vi "Init Tree.vi"(10 "Settings In":T4={"Step Values"=[], "Only Execute When Test Running"=TRUE, "Reset Sequence When Test Starts"=TRUE, "Current Sequence ID"=0, "Total Iterations"=0, "Current Step Start Timestamp"=0.0, "Number of Sequence Steps"=0, "Num of Analog Channels"=0, "Num of Digital Channels"=0, "Delay Before Starting Sequence"=0.0, "Show UI"=FALSE, "Time Remaining"=0.0, "Test Running"=FALSE, "Pause Timestamp"=0.0}, 11 "Init Refs":T3) -> (2 "Tree Data":cluster{string[], T1[]} {"?"."Data Type" items=["Tree Parent"=-1, "Numeric"=0, "String"=1, "Boolean"=2, "Enum"=3]}, 3 "Selected Tag":string)   [LabVIEW 2020, in "Sequencer with Output Values.lvlib" / "Sequencer with Output Values.lvclass"]
uses:
  Sequencer with Output Values.lvclass
  Params.ctl
  Step Settings.ctl
  Control Refs.ctl
  Tree Item Settings.ctl
  Data Type.ctl
  Global Tree Data.vi
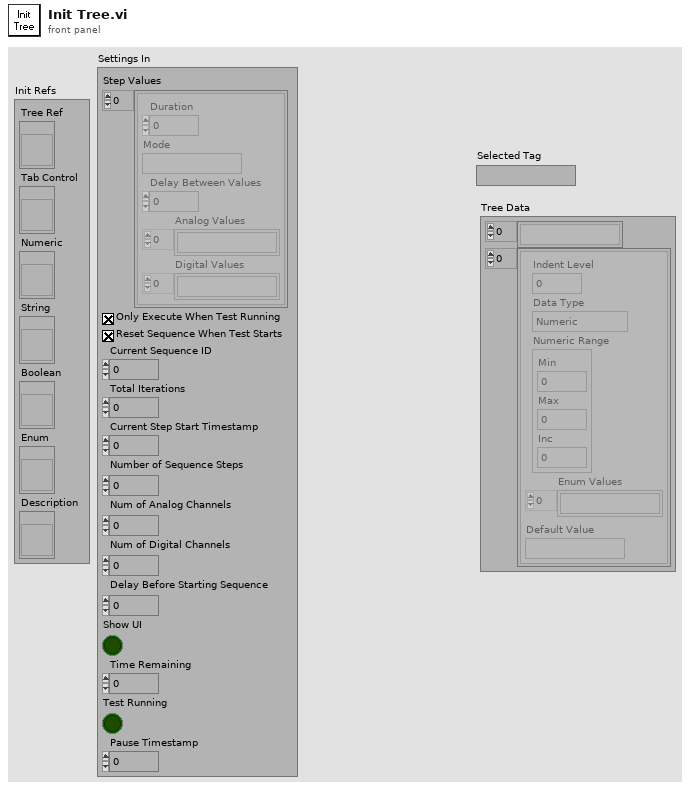
[diagram p1: front panel]
types:
  T1 = typedef "Sequencer with Output Values.lvlib/Sequencer with Output Values.lvclass/Tree Item Settings.ctl" = cluster{"Indent Level":i32, "Data Type":T2, "Numeric Range":cluster{"Min":dbl, "Max":dbl, "Inc":dbl}, "Enum Values":string[], "Default Value":string}
  T2 = typedef "Sequencer with Output Values.lvlib/Sequencer with Output Values.lvclass/Data Type.ctl" = i16
  T3 = typedef "Sequencer with Output Values.lvlib/Sequencer with Output Values.lvclass/Control Refs.ctl" = cluster{"Tree Ref":refnum<vi>, "Tab Control":refnum<vi>, "Numeric":refnum<vi>, "String":refnum<vi>, "Boolean":refnum<vi>, "Enum":refnum<vi>, "Description":refnum<vi>}
  T4 = typedef "Sequencer with Output Values.lvlib/Sequencer with Output Values.lvclass/Params.ctl" = cluster{"Step Values":T5[], "Only Execute When Test Running":bool, "Reset Sequence When Test Starts":bool, "Current Sequence ID":u32, "Total Iterations":u32, "Current Step Start Timestamp":dbl, "Number of Sequence Steps":i32, "Num of Analog Channels":i32, "Num of Digital Channels":i32, "Delay Before Starting Sequence":dbl, "Show UI":bool, "Time Remaining":dbl, "Test Running":bool, "Pause Timestamp":dbl}
  T5 = typedef "Sequencer with Output Values.lvlib/Sequencer with Output Values.lvclass/Step Settings.ctl" = cluster{"Duration":dbl, "Mode":string, "Delay Between Values":dbl, "Analog Values":string[], "Digital Values":string[]}
  T6 = cluster{"Left Cell String":string, "Child Text":string[], "Child Tag":string, "Item Indent":i32, "Child Only?":bool, "Glyph Index":i32}
  T7 = cluster{"Left Cell String":string, "Child Text":string[], "Child Tag":string, "Item Indent":i32, "Child Only?":bool, "Glyph Index":i32}[]
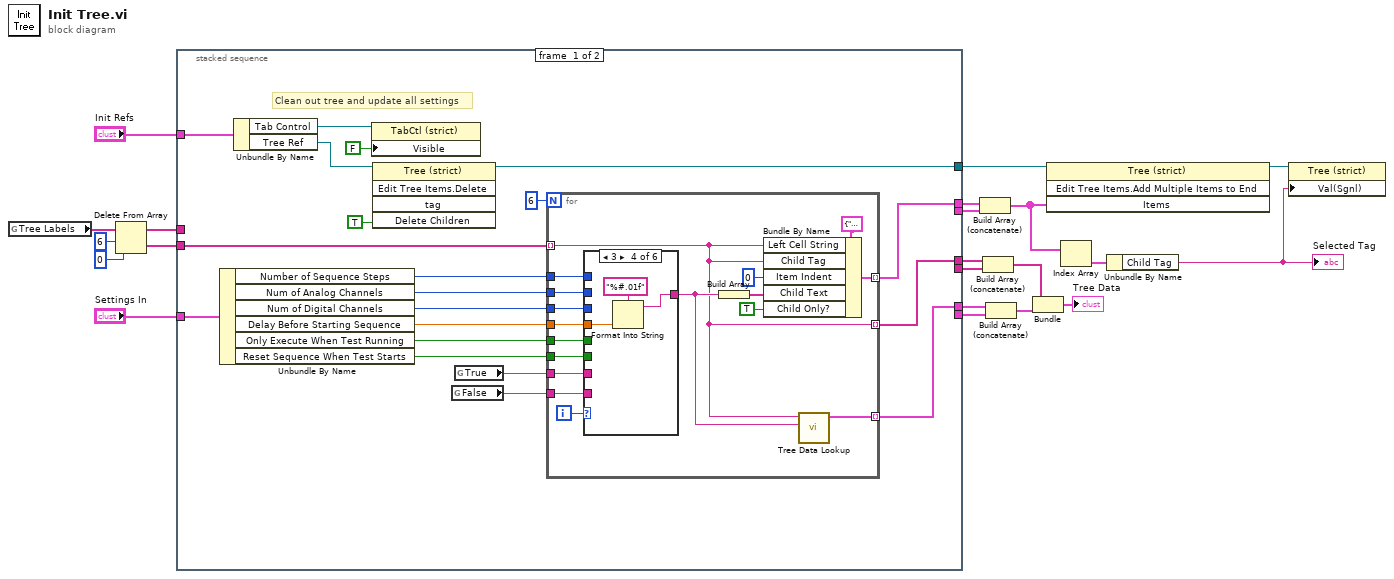
[diagram p0: block diagram]
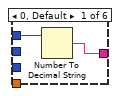
[diagram p2: hidden frame]
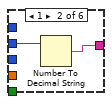
[diagram p3: hidden frame]
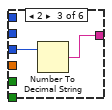
[diagram p4: hidden frame]
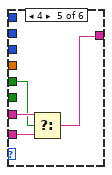
[diagram p5: hidden frame]
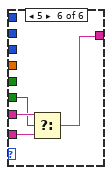
[diagram p6: hidden frame]
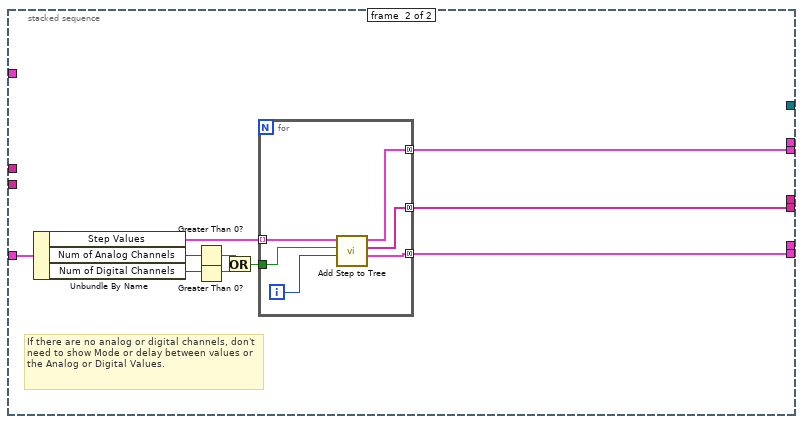
[diagram p7: hidden frame]
diagram:
  n1 = global read "Global Tree Data.vi" "Tree Labels"() -> (w16:string[])
  n2 = Delete From Array(array=w16, length=6, index=0) -> (deleted portion=w13:string[], array with subset deleted=w12:string[])
  n3 = stacked-sequence {
    tunnel: "Init Refs" -> [w39 _]
    tunnel: "Settings In" -> [w36 w85]
    tunnel: [_ w81] -> w18
    tunnel: [w26 _] -> w19
    tunnel: [w25 _] -> w17
    tunnel: w13 -> [w24 _]
    tunnel: w12 -> [_ _]
    tunnel: [w23 _] -> w7
    tunnel: [w22 _] -> w5
    tunnel: [_ w80] -> w2
    tunnel: [_ w79] -> w1
    frame #0 {
      # "Clean out tree and update all settings"
      n4 = Unbundle By Name(w36) -> ("Number of Sequence Steps"=w34:i32, "Num of Analog Channels"=w33:i32, "Num of Digital Channels"=w32:i32, "Delay Before Starting Sequence"=w31:dbl, "Only Execute When Test Running"=w30:bool, "Reset Sequence When Test Starts"=w29:bool)
      n5 = Unbundle By Name(w39) -> ("Tab Control"=w38:refnum<vi>, "Tree Ref"=w41:refnum<vi>)
      n6 = property class="TabCtl (strict)"(reference=w38, "Visible"=FALSE) -> ()  [unwired: 1 in, 2 out]
      n7 = invoke class="Tree (strict)" method="Edit Tree Items.Delete"(reference=w41, "Delete Children"=TRUE ("Delete Children?")) -> (reference out=w25:refnum<vi>)  [unwired: 3 in, 4 out]
      n8 = global read "Global Tree Data.vi" "False"() -> (w27:string)
      n9 = global read "Global Tree Data.vi" "True"() -> (w28:string)
      n10 = for {
        N: 6 -> [_]
        tunnel: w24 -> [w42] mode=indexing
        tunnel: w34 -> [w56]
        tunnel: w33 -> [w55]
        tunnel: w32 -> [w54]
        tunnel: w31 -> [w53]
        tunnel: w30 -> [w52]
        tunnel: w29 -> [w51]
        tunnel: w28 -> [w48]
        tunnel: w27 -> [w47]
        tunnel: [w46] -> w26 mode=indexing
        tunnel: [w43] -> w23 mode=indexing
        tunnel: [w42] -> w22 mode=indexing
        i -> [w49]
        n11 = case shown="3" w49 {
          tunnel: w56 -> [w60 _ _ _ _ _]
          tunnel: w55 -> [_ w62 _ _ _ _]
          tunnel: w54 -> [_ _ w64 _ _ _]
          tunnel: w53 -> [_ _ _ w66 _ _]
          tunnel: w52 -> [_ _ _ _ w69 _]
          tunnel: w51 -> [_ _ _ _ _ w72]
          tunnel: [w59 w61 w63 w65 w68 w73] -> w44
          tunnel: w48 -> [_ _ _ _ w71 w75]
          tunnel: w47 -> [_ _ _ _ w70 w74]
          frame 0, Default {
            n12 = Number To Decimal String(number=w60) -> (decimal integer string=w59:string)  [unwired: 1 in]
          }
          frame 1 {
            n13 = Number To Decimal String(number=w62) -> (decimal integer string=w61:string)  [unwired: 1 in]
          }
          frame 2 {
            n14 = Number To Decimal String(number=w64) -> (decimal integer string=w63:string)  [unwired: 1 in]
          }
          frame 3 {
            n15 = Format Into String(format string="%#.01f", w66) -> (resulting string=w65:string)  [unwired: 2 in, 1 out]
          }
          frame 4 {
            n16 = Select(t=w71, s=w69, f=w70) -> (s? t:f=w68:string)
          }
          frame 5 {
            n17 = Select(t=w75, s=w72, f=w74) -> (s? t:f=w73:string)
          }
        }
        n18 = Build Array(w44) -> (w50:string[])
        n19 = Bundle By Name(cluster=T6 {"Left Cell String"="", "Child Text"=[], "Child Tag"="", "Item Indent"=0, "Child Only?"=FALSE, "Glyph Index"=0} ("Item"), "Left Cell String"=w42, "Child Tag"=w42, "Item Indent"=0, "Child Text"=w50, "Child Only?"=TRUE) -> (w46:T6)
        n20 = call "Tree Data Lookup.vi"("Value"=w44, "Key"=w42) -> ("Tree Data"=w43:T1)  [unwired: 9 in]
      }
    }
    frame #1 {
      # "If there are no analog or digital channels, don't need to show Mode or delay between values or the Analog or Digital Values."
      n21 = Unbundle By Name(w85) -> ("Step Values"=w83:T5[], "Num of Analog Channels"=w84:i32, "Num of Digital Channels"=w82:i32)
      n22 = Greater Than 0?(x=w84) -> (x > 0?=w78:bool)
      n23 = Greater Than 0?(x=w82) -> (x > 0?=w77:bool)
      n24 = Or(x=w78, y=w77) -> (x .or. y?=w76:bool)
      n25 = for {
        tunnel: w83 -> [w91] mode=indexing
        tunnel: [w88] -> w81 mode=concatenating
        tunnel: [w87] -> w80 mode=concatenating
        tunnel: [w86] -> w79 mode=concatenating
        tunnel: w76 -> [w90]
        i -> [w89]
        n26 = call "Add Step to Tree.vi"("Step Index"=w89, "Channels Defined"=w90, "Step Settings"=w91) -> ("Tree Data"=w86:T1[], "Tree Tags"=w87:string[], "Tree Items"=w88:T7)  [unwired: 6 in]
      }
    }
  }
  n27 = Build Array (concatenate)(w19, w18) -> (w11:T7)
  n28 = Build Array (concatenate)(w5, w2) -> (w4:string[])
  n29 = Build Array (concatenate)(w7, w1) -> (w6:T1[])
  n30 = Bundle(w4, w6) -> (→"Tree Data":cluster{string[], T1[]})  [unwired: 1 in]
  n31 = invoke class="Tree (strict)" method="Edit Tree Items.Add Multiple Items to End"(reference=w17, "Items"=w11) -> (reference out=w9:refnum<vi>)  [unwired: 2 in, 3 out]
  n32 = Index Array(array=w11) -> (element=w10:T6)  [unwired: 1 in]
  n33 = Unbundle By Name(w10) -> ("Child Tag"=w8:string)
  "Selected Tag" <- w8
  n34 = property class="Tree (strict)"(reference=w9, "Val(Sgnl)"=w8) -> ()  [unwired: 1 in, 2 out]
